vi "Main-Get and Set Height.vi"() -> ()   [LabVIEW 2014]
uses:
  Main-Stage-PI/(Global) Current handle and LaserPower_YCC.vi
  <vilib>/DAQmx/create/channels.llb/DAQmx Create Channel (AI-Voltage-Basic).vi
  <vilib>/DAQmx/configure/timing.llb/DAQmx Timing (Sample Clock).vi
  <vilib>/DAQmx/read.llb/DAQmx Read (Analog 1D DBL 1Chan NSamp).vi
panel:
  out "Surface position (um)":dbl
  out "Stage Array Shift (nm)":dbl
  in  "Change power?":bool
  in  "Set power (mV)":dbl=1000.0
  in  "Filter type 2":T1(ring)=enum."Moving-window avg"
  out "inital Laser power":dbl
  out "Avg to Hz":dbl
  in  "Tab Control":enum32{"Raw QPDz-Stage", "Filtered QPDz-Stage"}(tab)
  out "Raw XY Graph":T2(graph)
  out "Filtered XY Graph":T2(graph)
  in  "Set Height":bool
  in  "Set Height (nm)":dbl=300.0
  in  "Avg points":i32=700
  out "traveling time (s)":dbl
  in  "Sampling Rate":dbl=32000.0 format="%0.2f"
  out "Position after move up":dbl
  in  "1/2 range  (um)":dbl=0.7000000000000001 format="%.3f"
  in  "scan rate  (um/s)":dbl=0.7 format="%.3f"
  out "Real Current Commanded position (um)":dbl=48.46734101118563 format="%0.5f"
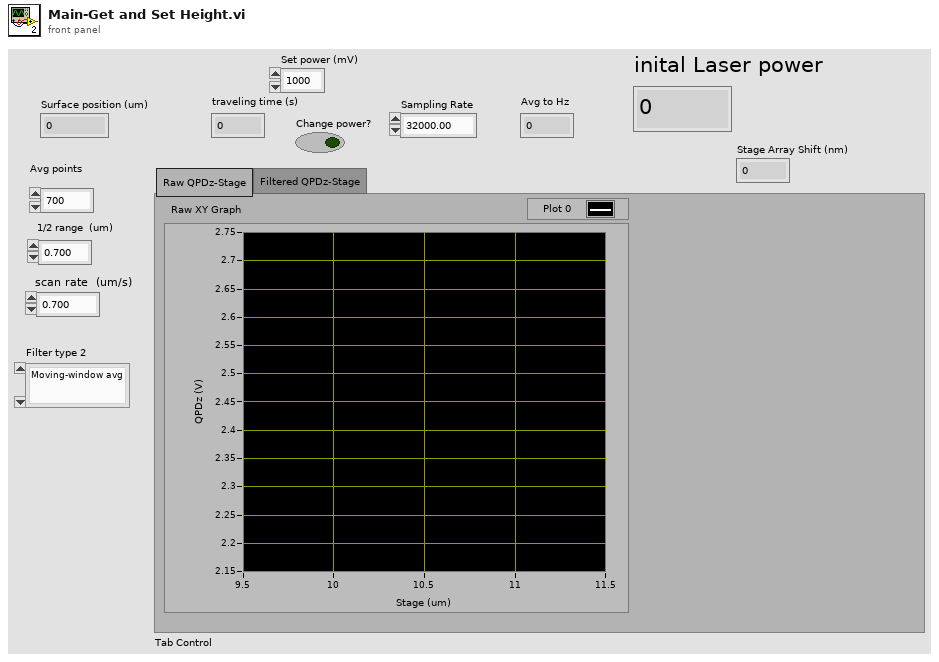
[diagram p1: front panel]
types:
  T1 = enum16{"Fixed-window avg", "Moving-window avg", "F+S-window avg", "S-G filter", "Fixed-window Median", "Moving-window Median "}
  T2 = cluster{"Filtered Stage Array":dbl[], "Filtered QPD data":dbl[]}
  T3 = cluster{"Correct Unfolded Stage Array (um)":dbl[], "Filtered QPD data":dbl[]}
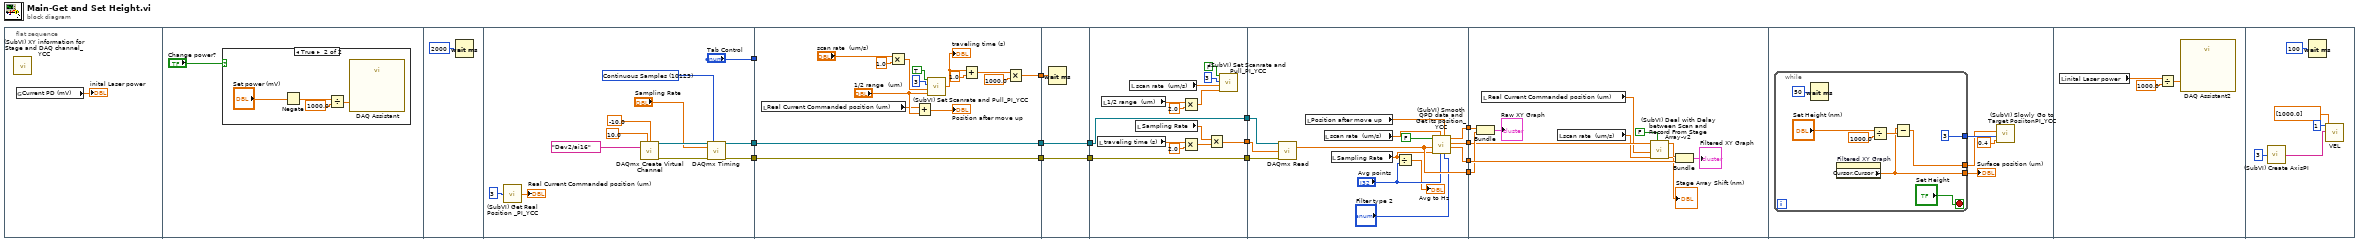
[diagram p0: block diagram]
diagram:
  n1 = flat-sequence {
    tunnel: [w25] -> w13
    tunnel: [w24] -> w9
    tunnel: ["Tab Control"] -> w1
    tunnel: [w44] -> w15
    tunnel: [w41] -> w14
    tunnel: w13 -> [w41]
    tunnel: [w40] -> w10
    tunnel: w9 -> [w40]
    tunnel: w1 -> [_]
    tunnel: w15 -> [w52]
    tunnel: w14 -> [w50]
    tunnel: [w51] -> w11
    tunnel: w10 -> [w51]
    tunnel: [w50] -> w7
    tunnel: [w62] -> w12
    tunnel: w11 -> [w62]
    tunnel: [w61] -> w8
    tunnel: w7 -> [w61]
    tunnel: [w59] -> w6
    tunnel: w12 -> [w79]
    tunnel: w8 -> [w78]
    tunnel: w6 -> [w77]
    tunnel: [w73] -> w5
    tunnel: [w72] -> w4
    tunnel: [w71] -> w3
    tunnel: [w70] -> w2
    tunnel: w5 -> [w85]
    tunnel: w4 -> [w90]
    tunnel: w3 -> [w89]
    tunnel: w2 -> [w88]
    frame #0 {
      n2 = call "(SubVI) XY information for Stage and DAQ channel_YCC.vi"() -> ()  [unwired: 4 in, 2 out]
      n3 = global read "(Global) Current handle and LaserPower_YCC.vi" "Current PD (mV)"() -> (→"inital Laser power":dbl)
    }
    frame #1 {
      n4 = case shown="True" "Change power?" {
        frame False {
        }
        frame True {
          n5 = Negate(x="Set power (mV)") -> (-x=w20:dbl)
          n6 = Divide(x=w20, y=1000.0) -> (x/y=w18:dbl)
          n7 = call "DAQ Assistant"("data"=w18) -> ()  [unwired: 17 in, 2 out]
        }
      }
    }
    frame #2 {
      n8 = Wait (ms)(milliseconds to wait=u32 2000) -> ()  [unwired: 1 out]
    }
    frame #3 {
      w27 = 10123 items=["Finite Samples"=10178, "Continuous Samples"=10123, "Hardware Timed Single Point"=12522] ("sample mode")
      n9 = call "(SubVI) Get Real Position _PI_YCC.vi"("Axis"=3) -> ("Real Current Commanded position (um)"=→"Real Current Commanded position (um)":dbl)  [unwired: 4 in]
      n10 = call-poly <vilib>:"DAQmx Create Virtual Channel.vi"("maximum value"=10.0, "minimum value"=-10.0, "physical channels"=tag "Dev2/ai16") -> ("task out"=w28:refnum<k21>, "error out"=w29:errorcluster)  [unwired: 11 in]
      n11 = call-poly <vilib>:"DAQmx Timing.vi"("task/channels in"=w28, "sample mode"=w27, "rate"="Sampling Rate", "error in"=w29) -> ("task out"=w25:refnum<k21>, "error out"=w24:errorcluster)  [unwired: 10 in]
    }
    frame #4 {
      n12 = local read "Real Current Commanded position (um)"() -> (w35:dbl)
      n13 = Multiply(x="scan rate  (um/s)", y=1.0) -> (x*y=w36:dbl)
      n14 = Add(x=w35, y="1/2 range  (um)") -> (x+y=→"Position after move up":dbl)
      n15 = call "(SubVI) Set Scanrate and Pull_PI_YCC.vi"("toward+ ?\nT=+, F=-"=TRUE ("toward+ ?\nT=+, F=-"), "axis"=u32 3, "scan rate  (um/s)"=w36, "range  (um)"="1/2 range  (um)") -> ("Traveling time (s)"=w39:dbl)  [unwired: 3 in, 1 out]
      "traveling time (s)" <- w39
      n16 = Add(x=w39, y=1.0) -> (x+y=w46:dbl)
      n17 = Multiply(x=w46, y=1000.0) -> (x*y=w44:dbl)
    }
    frame #5 {
      n18 = Wait (ms)(milliseconds to wait=w52) -> ()  [unwired: 1 out]
    }
    frame #6 {
      n19 = local read "traveling time (s)"() -> (w54:dbl)
      n20 = local read "1/2 range  (um)"() -> (w58:dbl)
      n21 = local read "scan rate  (um/s)"() -> (w63:dbl)
      n22 = local read "Sampling Rate"() -> (w60:dbl)
      n23 = Multiply(x=w58, y=2.0) -> (x*y=w56:dbl)
      n24 = Multiply(x=w54, y=2.0) -> (x*y=w53:dbl)
      n25 = Multiply(x=w60, y=w53) -> (x*y=w59:dbl)
      n26 = call "(SubVI) Set Scanrate and Pull_PI_YCC.vi"("toward+ ?\nT=+, F=-"=FALSE ("toward+ ?\nT=+, F=-"), "axis"=u32 3, "scan rate  (um/s)"=w63, "range  (um)"=w56) -> ()  [unwired: 3 in, 2 out]
    }
    frame #7 {
      n27 = call-poly <vilib>:"DAQmx Read.vi"("task/channels in"=w78, "number of samples per channel"=w77, "error in"=w79) -> ("data"=w70:dbl[])  [unwired: 10 in, 2 out]
      n28 = local read "Position after move up"() -> (w76:dbl)
      n29 = local read "scan rate  (um/s)"() -> (w75:dbl)
      n30 = local read "Sampling Rate"() -> (w69:dbl)
      n31 = Divide(x=w69, y="Avg points") -> (x/y=→"Avg to Hz":dbl)
      n32 = call "(SubVI) Smooth QPD data and Get its position_YCC.vi"("Filter type"="Filter type 2", "Initial position (um)"=w76, "Avg points"="Avg points", "scan rate  (um/s)"=w75, "Sampling rate (Hz)"=w69, "QPD data"=w70, "Direction\nT=+ \nF=-"=FALSE ("T=+ first\nF=- first")) -> ("Filtered QPD data"=w72:dbl[], "Filtered Stage Array"=w73:dbl[], "Raw Stage Array"=w71:dbl[])  [unwired: 2 in]
    }
    frame #8 {
      n33 = Bundle("Raw Stage Array"=w89, "data"=w88) -> (→"Raw XY Graph":cluster{"Raw Stage Array":dbl[], "data":dbl[]})  [unwired: 1 in]
      n34 = local read "Real Current Commanded position (um)"() -> (w83:dbl)
      n35 = local read "scan rate  (um/s)"() -> (w82:dbl)
      n36 = call "(SubVI) Deal with Delay between Scan and Record From Stage Array-v2.vi"("Toward first ?\nT=+, F=-"=FALSE ("Toward first ?\nT=+, F=-"), "Record scan rate  (um/s)"=w82, "Real initial position (um)"=w83, "Unfolded Stage Array (um)"=w85) -> ("Stage Array Shift (nm)"=→"Stage Array Shift (nm)":dbl, "Correct Unfolded Stage Array (um)"=w81:dbl[])  [unwired: 3 in, 1 out]
      n37 = Bundle("Correct Unfolded Stage Array (um)"=w81, "Filtered QPD data"=w90) -> (→"Filtered XY Graph":T3)  [unwired: 1 in]
    }
    frame #9 {
      n38 = while {
        tunnel: [w96] -> w93
        tunnel: [u32 3 ("axis")] -> w94
        tunnel: [w95] -> w91
        stop <- "Set Height" stop-if-true
        n39 = Wait (ms)(milliseconds to wait=u32 50) -> ()  [unwired: 1 out]
        n40 = property on="Filtered XY Graph" class="XYGraph (strict)"() -> ("Cursor.Cursor X"=w95:dbl)  [unwired: 2 in, 2 out]
        n41 = Divide(x="Set Height (nm)", y=1000.0) -> (x/y=w97:dbl)
        n42 = Subtract(x=w95, y=w97) -> (x-y=w96:dbl)
      }
      "Surface position (um)" <- w91
      n43 = call "(SubVI) Slowly Go to Target PosiitonPI_YCC.vi"("scan rate  (um/s)"=0.4, "axis"=w94, "Target position (um)"=w93) -> ()  [unwired: 4 in, 1 out]
    }
    frame #10 {
      n44 = local read "inital Laser power"() -> (w105:dbl)
      n45 = Divide(x=w105, y=1000.0) -> (x/y=w103:dbl)
      n46 = call "DAQ Assistant2"("data"=w103) -> ()  [unwired: 17 in, 2 out]
    }
    frame #11 {
      n47 = call "(SubVI) Create AxisPI.vi"("axis"=u32 3) -> ("Axis String Array"=w107:string[])  [unwired: 2 in, 2 out]
      n48 = Wait (ms)(milliseconds to wait=u32 100) -> ()  [unwired: 1 out]
      n49 = call "VEL.vi"("System no."=1, "Axes to set"=w107, "Velocity values"=dbl[] [1000.0]) -> ()  [unwired: 3 in, 14 out]
    }
  }
